vi "Constants.vi"() -> ()   [LabVIEW 2023, in "Embedded TDMS Logger Shared.lvlib"]
doc: "Use this Global VI to access the GUIDs assigned to the page resources of the Custom Device."
uses:
  Embedded TDMS Logger Shared.lvlib
panel:
  in  "Tab Control":enum32{"GUIDs", "Constants", "Properties"}(tab)
  in  "Waveform Channel Level":string="d4831e4e-4340-44f6-a949-9831e2f55b5e"
  in  "Channel Level":string="22f26562-5b63-4f30-88d3-24dae5cd9a1b"
  in  "Group Level":string="ad36ff05-e498-4721-9ffb-d3fa67663aa8"
  in  "Embedded TDMS Logger":string="daea7e29-2fc3-47a8-981c-469a5cb8af3b"
  in  "Compiled.Settings":string="Compiled.Settings"
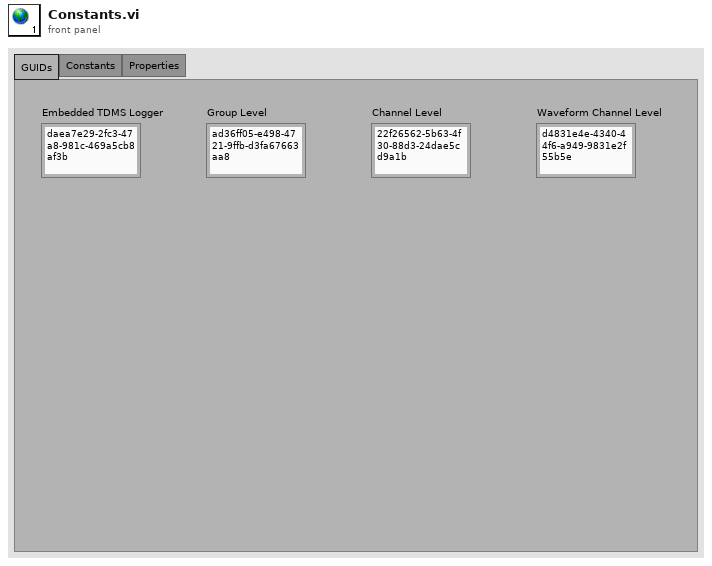
[diagram p1: front panel]
diagram:
